vi "measure-tunnelling(SubVI).vi"(0 ".NET引用句柄输入":refnum<k24>, 1 "error":refnum<queue>, 5 "Timeout (20000 ms)":u32=20000, 7 "Resource In":refnum<visa-resource-name>, 9 "scan current":bool, 11 "error in (no error)":errorcluster, 12 "ch str":string) -> (4 "data":string[](array[string]), 8 "Numeric":sgl, 15 "error out":errorcluster)   [LabVIEW 2019]
uses:
  lib/QDInstrument.dll
  ppms-6621&2182-7001 tunnelling/Keithley 622x/Configure/Format/Typedefs/KE622x -- Optional Meas Elements.ctl
  ppms-6621&2182-7001 tunnelling/KE7001.LLB/Keith 7001 Open/Close Chan.vi
  ppms-6621&2182-7001 tunnelling/SubVI.lvlib
  ppms-6621&2182-7001 tunnelling/Keithley 622x/Keithley 622x.lvlib
panel:
  out "Timeout? 2":bool
  out "Execution Time 2":dbl
  out "array w/ subset deleted 2":sgl[](array[numeric])
  out "element 2":bool
  out "array w/ subset deleted":sgl[](array[numeric])
  out "element":bool
  out "Execution Time":dbl
  out "Timeout?":bool
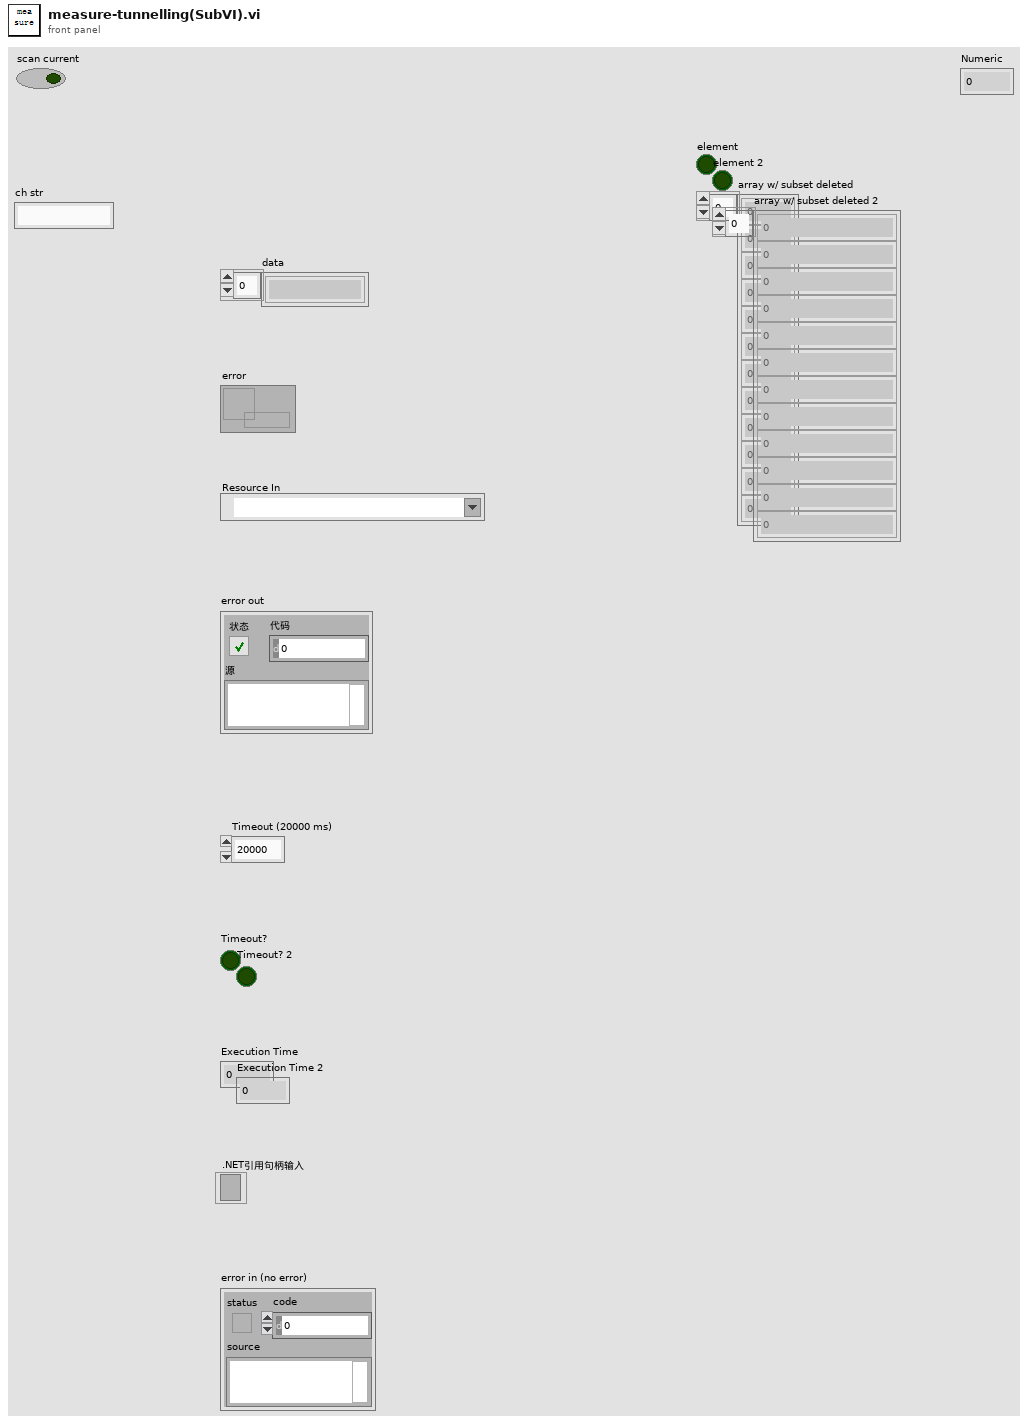
[diagram p1: front panel]
types:
  T1 = cluster{"slot/memory":i16, "channel/row":i16, "column":i16, bool, bool}[]
  T2 = typedef "Keithley 622x.lvlib/KE622x -- Optional Meas Elements.ctl" = cluster{"Timstamp?":bool, "Reading Num?":bool, "Source Value?":bool, "Compliance?":bool, "Average Voltage?":bool}
  T3 = cluster{"error":bool, "code":i32, "source":string}
  T4 = typedef "Keithley 622x.lvlib/KE622x -- Meas Event Reg State.ctl" = cluster{"B0, ROF:  KE2182A Delta Reading Overflow Event?":bool, "B1, Int:  Interlock OK Event?":bool, "B2, Temp:  Over Temperature Event?":bool, "B3, Comp:  Compliance Event?":bool, "B5, RAV:  Delta Reading Available Event?":bool, "B6, TN:  User Defined Reading Number Stored In Buffer Event?":bool, "B7, BAV:  At Least 2 Readings Stored In Buffer Event?":bool, "B12, BQF:  Buffer Quarter Full Event?":bool, "B8, BHF:  Buffer Half Full Event?":bool, "B13, B3QF:  Buffer 3/4 Full Event?":bool, "B9, BFL:  Buffer Full Event?":bool}
  T5 = typedef "Keithley 622x.lvlib/KE622x -- Trace Buf.ctl" = cluster{"Additional Valid Arrays":T2, "Reading Num":u32[], "Timestamp (secs)":sgl[], "Source Val (A)":sgl[], "Reading":sgl[], "Average Voltage (V)":sgl[], "Compliance?":bool[]}
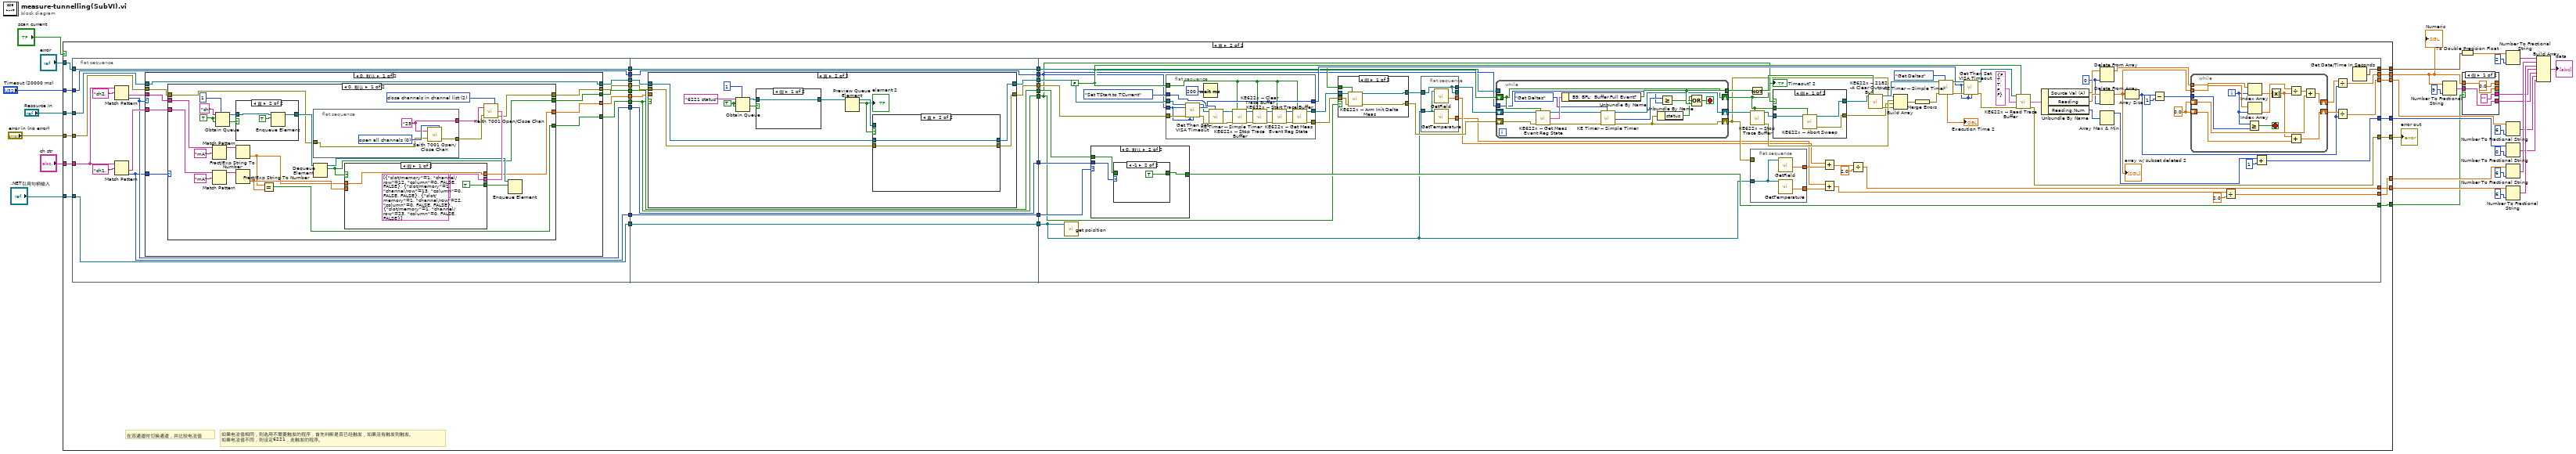
[diagram p0: block diagram]
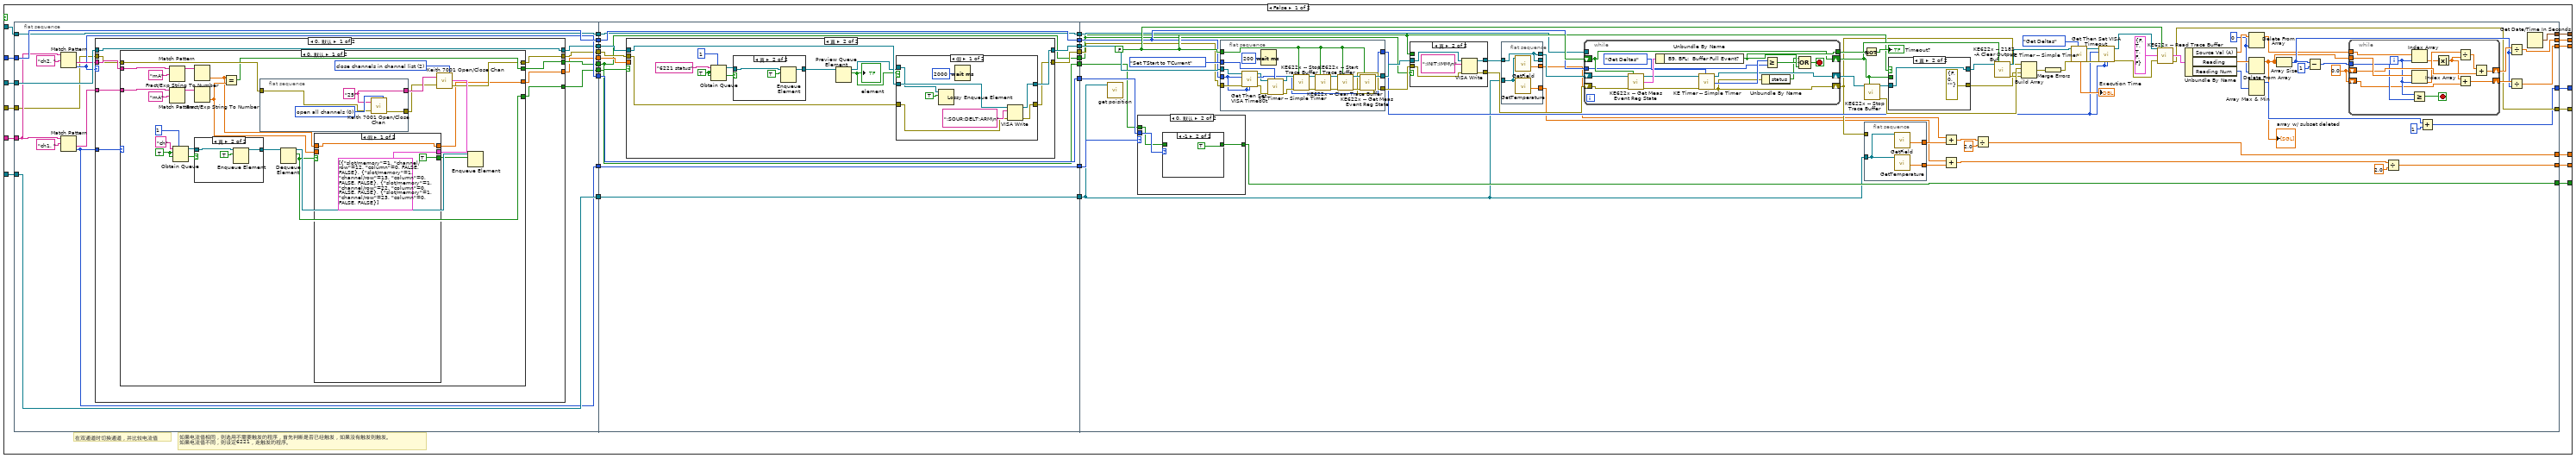
[diagram p2: hidden frame]
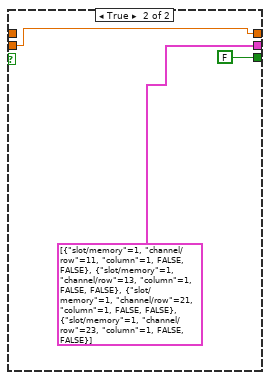
[diagram p4: hidden frame]
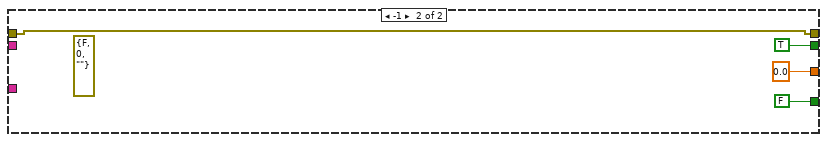
[diagram p5: hidden frame]
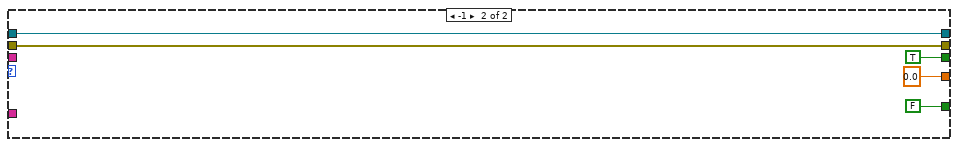
[diagram p6: hidden frame]
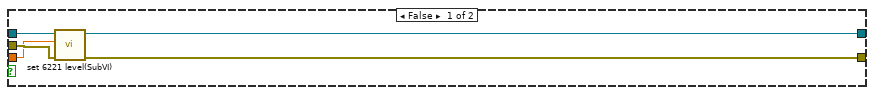
[diagram p7: hidden frame]
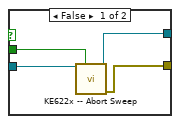
[diagram p10: hidden frame]
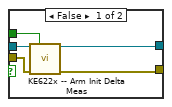
[diagram p11: hidden frame]
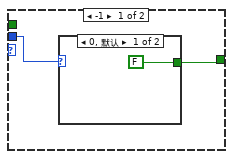
[diagram p12: hidden frame]
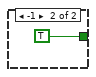
[diagram p13: hidden frame]
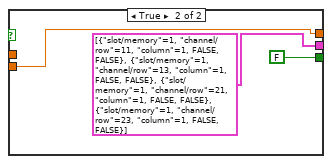
[diagram p16: hidden frame]
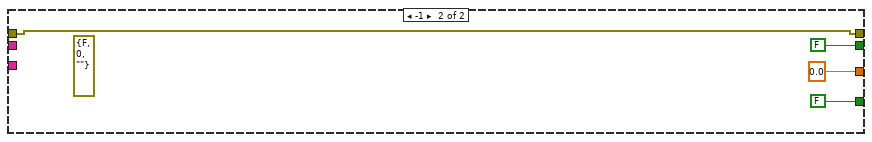
[diagram p17: hidden frame]
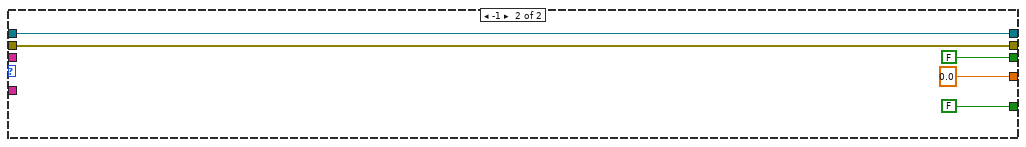
[diagram p18: hidden frame]
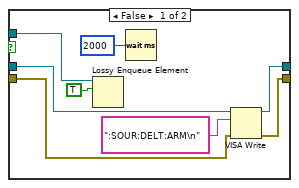
[diagram p20: hidden frame]
diagram:
  n1 = case shown="真" "scan current" {
    tunnel: [w45 w342] -> w31
    tunnel: ".NET引用句柄输入" -> [w44 w330]
    tunnel: "Resource In" -> [w43 w341]
    tunnel: "error in (no error)" -> [w42 w340]
    tunnel: "Timeout (20000 ms)" -> [w41 w339]
    tunnel: "error" -> [w40 w329]
    tunnel: [w39 w338] -> w25
    tunnel: [w38 w337] -> w22
    tunnel: [w37 w336] -> w19
    tunnel: [w36 w335] -> w9
    tunnel: "ch str" -> [w35 w334]
    tunnel: [w34 w333] -> w7
    tunnel: [w33 w332] -> w6
    tunnel: [w32 w331] -> w2
    frame False {
      # "如果电流值相同，则选用不需要触发的程序，首先判断是否已经触发，如果没有触发则触发。\n如果电流值不同，则设定6221，走触发的程序。"
      # "在双通道时切换通道，并比较电流值"
      n2 = flat-sequence {
        tunnel: w40 -> [w79]
        tunnel: w41 -> [w80]
        tunnel: w42 -> [w69]
        tunnel: w43 -> [w76]
        tunnel: w44 -> [w81]
        tunnel: [w81] -> w64
        tunnel: [w80] -> w63
        tunnel: [w79] -> w62
        tunnel: w35 -> [w75]
        tunnel: [w72] -> w61
        tunnel: [w71] -> w60
        tunnel: [w70] -> w59
        tunnel: [w68] -> w58
        tunnel: [w67] -> w57
        tunnel: [w66] -> w56
        tunnel: [w65] -> w55
        tunnel: w64 -> [w150]
        tunnel: [w150] -> w54
        tunnel: w63 -> [w149]
        tunnel: [w149] -> w53
        tunnel: w62 -> [w148]
        tunnel: [w148] -> w52
        tunnel: w61 -> [w147]
        tunnel: [w147] -> w51
        tunnel: w60 -> [w146]
        tunnel: [w146] -> w50
        tunnel: w59 -> [w145]
        tunnel: [w145] -> w49
        tunnel: w58 -> [w139]
        tunnel: w57 -> [w144]
        tunnel: w56 -> [w143]
        tunnel: w55 -> [w142]
        tunnel: [w141] -> w48
        tunnel: [w140] -> w47
        tunnel: [w139] -> w46
        tunnel: [w187] -> w38
        tunnel: [w188] -> w37
        tunnel: [w201] -> w45
        tunnel: [w224] -> w34
        tunnel: [w207] -> w36
        tunnel: [w219] -> w33
        tunnel: [w218] -> w39
        tunnel: w54 -> [w199]
        tunnel: w53 -> [w216]
        tunnel: w52 -> [w215]
        tunnel: [w206] -> w32
        tunnel: w51 -> [w205]
        tunnel: w50 -> [w204]
        tunnel: w49 -> [w203]
        tunnel: w48 -> [w217]
        tunnel: w47 -> [w228]
        tunnel: w46 -> [w202]
        frame #0 {
          n3 = Match Pattern(string=w75, regular expression="ch2, " ("正则表达式")) -> (after substring=w73:string, offset past match=w72:i32)  [unwired: 1 in, 2 out]
          n4 = Match Pattern(string=w75, regular expression="ch1, " ("正则表达式")) -> (after substring=w74:string, offset past match=w71:i32)  [unwired: 1 in, 2 out]
          n5 = case shown="0, 默认" w72 {
            tunnel: w76 -> [w82 w136]
            tunnel: w74 -> [w90 _]
            tunnel: w73 -> [w89 _]
            tunnel: w71 -> [w88 _]
            tunnel: [w87 FALSE ("create if not found? (T)")] -> w70
            tunnel: w69 -> [w86 w137]
            tunnel: [w85 TRUE] -> w68
            tunnel: [w84 w137] -> w67
            tunnel: [w83 0.0] -> w66
            tunnel: [w82 w136] -> w65
            frame 0, Default {
              n6 = case shown="0, 默认" w88 {
                tunnel: w90 -> [w101 _]
                tunnel: w89 -> [w111 _]
                tunnel: [w103 FALSE ("create if not found? (T)")] -> w87
                tunnel: w86 -> [w97 w131]
                tunnel: [w94 TRUE] -> w85
                tunnel: [w93 w131] -> w84
                tunnel: [w92 0.0] -> w83
                frame 0, Default {
                  w109 = TRUE ("create if not found? (T)")
                  w114 = u16 2 items=["open all channels", "open channels in channel list", "close channels in channel list"] ("open/close (open all:0)")
                  n7 = Match Pattern(string=w111, regular expression="mA" ("正则表达式")) -> (before substring=w98:string)  [unwired: 1 in, 3 out]
                  n8 = Match Pattern(string=w101, regular expression="mA" ("正则表达式")) -> (before substring=w99:string)  [unwired: 1 in, 3 out]
                  n9 = Obtain Queue(max queue size (-1, unlimited)=1, name (unnamed)="ch", element data type=w109, create if not found? (T)=w109) -> (queue out=w107:refnum<queue>, created new?=w108:bool)  [unwired: 1 in, 1 out]
                  n10 = Fract/Exp String To Number(string=w98) -> (number=w95:dbl)  [unwired: 3 in, 1 out]
                  n11 = Fract/Exp String To Number(string=w99) -> (number=w96:dbl)  [unwired: 3 in, 1 out]
                  n12 = case shown="真" w108 {
                    tunnel: w107 -> [w116 w119]
                    tunnel: [w116 w117] -> w106
                    frame False {
                    }
                    frame True {
                      n13 = Enqueue Element(queue=w119, element=TRUE) -> (queue out=w117:refnum<queue>)  [unwired: 2 in, 2 out]
                    }
                  }
                  n14 = Equal?(x=w95, y=w96) -> (x = y?=w94:bool)
                  n15 = flat-sequence {
                    tunnel: [w122] -> w115
                    tunnel: [w121] -> w112
                    tunnel: w97 -> [w120]
                    frame #0 {
                      w123 = u16 0 items=["open all channels", "open channels in channel list", "close channels in channel list"] ("open/close (open all:0)")
                      w122 = "25" ("GPIB address")
                      n16 = call "Keith 7001 Open/Close Chan.vi"("GPIB address"=w122, "error in"=w120, "open/close (open all:0)"=w123) -> ("error out"=w121:T3)  [unwired: 1 in]
                    }
                  }
                  n17 = Dequeue Element(queue=w106) -> (queue out=w105:refnum<queue>, element=w103:bool)  [unwired: 2 in, 2 out]
                  n18 = case shown="假" w103 {
                    tunnel: [T1 [{"slot/memory"=1, "channel/row"=12, "column"=0, FALSE, FALSE}, {"slot/memory"=1, "channel/row"=13, "column"=0, FALSE, FALSE}, {"slot/memory"=1, "channel/row"=22, "column"=0, FALSE, FALSE}, {"slot/memory"=1, "channel/row"=23, "column"=0, FALSE, FALSE}] ("channel list") T1 [{"slot/memory"=1, "channel/row"=11, "column"=1, FALSE, FALSE}, {"slot/memory"=1, "channel/row"=13, "column"=1, FALSE, FALSE}, {"slot/memory"=1, "channel/row"=21, "column"=1, FALSE, FALSE}, {"slot/memory"=1, "channel/row"=23, "column"=1, FALSE, FALSE}] ("channel list")] -> w113
                    tunnel: [TRUE FALSE] -> w104
                    tunnel: w96 -> [_ w128]
                    tunnel: w95 -> [w124 _]
                    tunnel: [w124 w128] -> w92
                    frame False {
                    }
                    frame True {
                    }
                  }
                  n19 = call "Keith 7001 Open/Close Chan.vi"("GPIB address"=w115, "error in"=w112, "open/close (open all:0)"=w114, "channel list"=w113) -> ("error out"=w93:T3)
                  n20 = Enqueue Element(queue=w105, element=w104) -> ()  [unwired: 2 in, 3 out]
                }
                frame -1 {
                  (unwired) errorcluster {"status"=FALSE, "code"=0, "source"=""} ("错误输出")
                }
              }
            }
            frame -1 {
            }
          }
        }
        frame #1 {
          n21 = case shown="真" w139 {
            tunnel: w144 -> [w155 w162]
            tunnel: w143 -> [w154 _]
            tunnel: w142 -> [w153 w163]
            tunnel: [w152 w161] -> w140
            tunnel: [w151 w160] -> w141
            frame False {
              n22 = call "set 6221 level(SubVI).vi"("错误输入（无错误）"=w155, "电流（mA）"=w154, "VISA引用句柄输入"=w153) -> ("错误输出"=w151:errorcluster, "VISA引用句柄输出"=w152:refnum<visa-resource-name>)  [unwired: 7 in]
            }
            frame True {
              w164 = TRUE ("create if not found? (T)")
              n23 = Obtain Queue(max queue size (-1, unlimited)=1, name (unnamed)="6221 status", element data type=w164, create if not found? (T)=w164) -> (queue out=w166:refnum<queue>, created new?=w167:bool)  [unwired: 1 in, 1 out]
              n24 = case shown="真" w167 {
                tunnel: w166 -> [w178 w181]
                tunnel: [w178 w179] -> w159
                frame False {
                }
                frame True {
                  n25 = Enqueue Element(queue=w181, element=TRUE) -> (queue out=w179:refnum<queue>)  [unwired: 2 in, 2 out]
                }
              }
              n26 = Preview Queue Element(queue=w159) -> (queue out=w158:refnum<queue>, element=w157:bool)  [unwired: 2 in, 2 out]
              "element" <- w157
              n27 = case shown="假" w157 {
                tunnel: w158 -> [w170 _]
                tunnel: w163 -> [w171 w176]
                tunnel: [w172 w176] -> w161
                tunnel: w162 -> [w174 w177]
                tunnel: [w173 w177] -> w160
                frame False {
                  n28 = Lossy Enqueue Element(queue=w170, element=TRUE) -> ()  [unwired: 1 in, 4 out]
                  n29 = Wait (ms)(milliseconds to wait=u32 2000) -> ()  [unwired: 1 out]
                  n30 = VISA Write(VISA resource name=w171, write buffer=":SOUR:DELT:ARM\n" ("format string"), error in (no error)=w174) -> (VISA resource name out=w172:refnum<visa-resource-name>, error out=w173:errorcluster)  [unwired: 1 out]
                }
                frame True {
                }
              }
            }
          }
        }
        frame #2 {
          w227 = FALSE ("Check For SCPI Errors? (T) 2")
          w184 = 0 ("index")
          w222 = sgl 0.0 ("Numeric")
          n31 = call "get poisition.vi"("Instrument Ref In"=w199) -> ()  [unwired: 4 in, 3 out]
          n32 = case shown="0, 默认" w204 {
            tunnel: [w293 w298] -> w206
            tunnel: w205 -> [w292 w297]
            tunnel: w203 -> [_ w296]
            frame -1 {
              n33 = case shown="0, 默认" w292 {
                tunnel: [FALSE TRUE] -> w293
                frame 0, Default {
                }
                frame -1 {
                }
              }
            }
            frame 0, Default {
              n34 = case shown="-1" w297 {
                tunnel: [w299 TRUE] -> w298
                tunnel: w296 -> [w299 _]
                frame 0, Default {
                }
                frame -1 {
                }
              }
            }
          }
          n35 = flat-sequence {
            tunnel: enum16{"Set TStart to TCurrent", "Get Deltas"}."Set TStart to TCurrent" ("Action") -> [w264]
            tunnel: [w261] -> w237
            tunnel: [w260] -> w236
            tunnel: [w257] -> w229
            tunnel: w228 -> [w254]
            tunnel: w227 -> [w253]
            tunnel: w217 -> [w252]
            tunnel: w216 -> [w251]
            frame #0 {
              n36 = call "Get Then Set VISA Timeout.vi"("VISA Resource Name In"=w254, "New Timeout (msecs)"=w251, "error in (no error)"=w252, "Max Timeout (300 secs)"=w251, "Min Timeout (3 secs)"=w251) -> ("VISA Resource Name Out (dupl)"=w256:refnum<visa-resource-name>, "Old Timeout (msecs)"=w257:u32, "error out"=w255:errorcluster)  [unwired: 7 in, 1 out]
              n37 = Wait (ms)(milliseconds to wait=u32 200) -> ()  [unwired: 1 out]
              n38 = call "KE Timer -- Simple Timer.vi"("Resource In"=w256, "error in (no error)"=w255, "Action"=w264) -> ("Resource Out (dupl)"=w263:refnum<visa-resource-name>, "error out (dupl)"=w262:errorcluster)  [unwired: 7 in, 8 out]
              n39 = call "KE622x -- Stop Trace Buffer.vi"("Resource In"=w263, "Check For SCPI Errors? (T)"=w253, "error in (no error)"=w262) -> ("Resource Out (dupl)"=w268:refnum<visa-resource-name>, "error out"=w267:errorcluster)  [unwired: 11 in]
              n40 = call "KE622x -- Clear Trace Buffer.vi"("Resource In"=w268, "Check For SCPI Errors? (T)"=w253, "error in (no error)"=w267) -> ("Resource Out (dupl)"=w259:refnum<visa-resource-name>, "error out"=w258:errorcluster)  [unwired: 11 in]
              n41 = call "KE622x -- Start Trace Buffer.vi"("Resource In"=w259, "Check For SCPI Errors? (T)"=w253, "error in (no error)"=w258) -> ("Resource Out (dupl)"=w265:refnum<visa-resource-name>, "error out"=w266:errorcluster)  [unwired: 11 in]
              n42 = call "KE622x -- Get Meas Event Reg State.vi"("VISA Resource In"=w265, "Error Query (T)?"=w253, "error in (no error)"=w266) -> ("VISA Resource Out (dupl)"=w261:refnum<visa-resource-name>, "error out"=w260:errorcluster)  [unwired: 10 in, 1 out]
            }
          }
          n43 = case shown="真" w202 {
            tunnel: [w286 w288] -> w244
            tunnel: [w285 w287] -> w198
            tunnel: w237 -> [w282 w290]
            tunnel: w236 -> [w284 w289]
            tunnel: w227 -> [w283 _]
            frame False {
              n44 = call "KE622x -- Arm Init Delta Meas.vi"("Resource In"=w282, "Check For SCPI Errors? (T)"=w283, "error in (no error)"=w284) -> ("Resource Out (dupl)"=w285:refnum<visa-resource-name>, "error out"=w286:errorcluster)  [unwired: 11 in]
            }
            frame True {
              n45 = VISA Write(VISA resource name=w290, write buffer=":INIT:IMM\n", error in (no error)=w289) -> (VISA resource name out=w287:refnum<visa-resource-name>, error out=w288:errorcluster)  [unwired: 1 out]
            }
          }
          n46 = flat-sequence {
            tunnel: w199 -> [w270]
            tunnel: [w272] -> w193
            tunnel: [w271] -> w196
            tunnel: w198 -> [w269]
            tunnel: [w269] -> _
            tunnel: [w269] -> w197
            frame #0 {
              n47 = call "GetField.vi"("Instrument Ref In"=w270) -> ("Field"=w271:dbl)  [unwired: 4 in, 4 out]
              n48 = call "GetTemperature.vi"("Instrument Ref In"=w270) -> ("Temperature"=w272:dbl)  [unwired: 4 in, 4 out]
            }
          }
          n49 = while {
            shift-right: [w303] -> w200
            shift-left: w244 -> [w315]
            shift-right: [w305] -> w241
            shift-left: w197 -> [w314]
            tunnel: [w307] -> w243
            shift-right: [w304] -> w213
            shift-left: w227 -> [w304]
            tunnel: w216 -> [w301]
            tunnel: w215 -> [_]
            stop <- w308 stop-if-true
            n50 = call "KE622x -- Get Meas Event Reg State.vi"("VISA Resource In"=w314, "Error Query (T)?"=w304, "error in (no error)"=w315) -> ("VISA Resource Out (dupl)"=w311:refnum<visa-resource-name>, "KE622x Meas Event Reg"=w313:T4, "error out"=w312:errorcluster)  [unwired: 10 in]
            n51 = Unbundle By Name(w313) -> ("B9, BFL:  Buffer Full Event?"=w307:bool)
            n52 = call "KE Timer -- Simple Timer.vi"("Resource In"=w311, "error in (no error)"=w312, "Action"=enum16{"Set TStart to TCurrent", "Get Deltas"}."Get Deltas") -> ("Resource Out (dupl)"=w305:refnum<visa-resource-name>, "TCurrent - TStart (ms)"=w309:u32, "error out (dupl)"=w303:errorcluster)  [unwired: 7 in, 7 out]
            n53 = Unbundle By Name(w303) -> ("status"=w302:bool)
            n54 = Greater Or Equal?(x=w309, y=w301) -> (x >= y?=w306:bool)
            n55 = Compound Arithmetic op=OR(w302, w306, w307) -> (w308:bool)
          }
          n56 = Not(x=w243) -> (.not. x?=→"Timeout?":bool)
          n57 = call "KE622x -- Stop Trace Buffer.vi"("Resource In"=w241, "Check For SCPI Errors? (T)"=w213) -> ("Resource Out (dupl)"=w214:refnum<visa-resource-name>, "error out"=w234:errorcluster)  [unwired: 12 in]
          n58 = flat-sequence {
            tunnel: w199 -> [w273]
            tunnel: [w275] -> w194
            tunnel: [w274] -> w195
            tunnel: w200 -> [_]
            frame #0 {
              n59 = call "GetField.vi"("Instrument Ref In"=w273) -> ("Field"=w274:dbl)  [unwired: 4 in, 4 out]
              n60 = call "GetTemperature.vi"("Instrument Ref In"=w273) -> ("Temperature"=w275:dbl)  [unwired: 4 in, 4 out]
            }
          }
          n61 = case shown="真" w202 {
            tunnel: w213 -> [w278 _]
            tunnel: [w277 w281] -> w212
            tunnel: [w276 errorcluster {"status"=FALSE, "code"=0, "source"=""} ("error out")] -> w211
            tunnel: w214 -> [w279 w281]
            frame False {
              n62 = call "KE622x -- Abort Sweep.vi"("Resource In"=w279, "Check For SCPI Errors? (T)"=w278) -> ("Resource Out (dupl)"=w277:refnum<visa-resource-name>, "error out"=w276:errorcluster)  [unwired: 12 in]
            }
            frame True {
            }
          }
          n63 = Add(x=w196, y=w195) -> (x+y=w191:dbl)
          n64 = Add(x=w193, y=w194) -> (x+y=w192:dbl)
          n65 = Divide(x=w191, y=2.0) -> (x/y=w188:dbl)
          n66 = call "KE622x -- 2182 -A Clear Output Buf.vi"("622x Resource In"=w212, "Check For SCPI Errors? (T)"=w213) -> ("622x Resource Out (dupl)"=w240:refnum<visa-resource-name>, "error out"=w233:errorcluster)  [unwired: 11 in, 1 out]
          n67 = Build Array(w200, w234, w211, w233) -> (w235:errorcluster[])
          n68 = Merge Errors(w235) -> (w232:errorcluster)
          n69 = call "KE Timer -- Simple Timer.vi"("Resource In"=w240, "error in (no error)"=w232, "Action"=enum16{"Set TStart to TCurrent", "Get Deltas"}."Get Deltas") -> ("TCurrent - TStart (s)"=→"Execution Time":dbl, "Resource Out (dupl)"=w230:refnum<visa-resource-name>, "error out (dupl)"=w231:errorcluster)  [unwired: 7 in, 7 out]
          n70 = call "Get Then Set VISA Timeout.vi"("VISA Resource Name In"=w230, "New Timeout (msecs)"=w229, "error in (no error)"=w231, "Max Timeout (300 secs)"=w229, "Min Timeout (3 secs)"=w229) -> ("VISA Resource Name Out (dupl)"=w226:refnum<visa-resource-name>, "error out"=w225:errorcluster)  [unwired: 7 in, 2 out]
          n71 = call "KE622x -- Read Trace Buffer.vi"("Resource In"=w226, "Check For SCPI Errors? (T)"=w227, "Meas Elements To Return"=T2 {"Timstamp?"=FALSE, "Reading Num?"=TRUE, "Source Value?"=TRUE, "Compliance?"=FALSE, "Average Voltage?"=FALSE}, "error in (no error)"=w225) -> ("Trace Buf"=w249:T5, "error out"=w218:errorcluster)  [unwired: 9 in, 1 out]
          n72 = Unbundle By Name(w249) -> ("Source Val (A)"=w185:sgl[], "Reading"=w186:sgl[], "Reading Num"=w223:u32[])
          n73 = Delete From Array(array=w185, index=w184) -> (array with subset deleted=w183:sgl[])  [unwired: 1 in, 1 out]
          n74 = Delete From Array(array=w186, index=w184) -> (array with subset deleted=w182:sgl[])  [unwired: 1 in, 1 out]
          "array w/ subset deleted" <- w182
          n75 = Array Max & Min(array=w223) -> (max value=w209:u32)  [unwired: 3 out]
          n76 = Array Size(array=w182) -> (size(s)=w220:i32)
          n77 = Subtract(x=w220, y=1) -> (x-y=w246:i32)
          n78 = while {
            tunnel: w182 -> [w328]
            shift-right: [w326] -> w248
            shift-left: w222 -> [w327]
            tunnel: w246 -> [w325]
            tunnel: w183 -> [w323]
            shift-right: [w320] -> w221
            shift-left: w222 -> [w321]
            i -> [w322]
            stop <- w324 stop-if-true
            n79 = Greater Or Equal?(x=w322, y=w325) -> (x >= y?=w324:bool)
            n80 = Index Array(array=w323, index=w322) -> (element=w318:sgl)
            n81 = Index Array(array=w328, index=w322) -> (element=w319:sgl)
            n82 = Absolute Value(x=w318) -> (abs(x)=w316:sgl)
            n83 = Divide(x=w319, y=w316) -> (x/y=w317:sgl)
            n84 = Add(x=w316, y=w321) -> (x+y=w320:sgl)
            n85 = Add(x=w317, y=w327) -> (x+y=w326:sgl)
          }
          n86 = Divide(x=w192, y=2.0) -> (x/y=w187:dbl)
          n87 = Add(x=w209, y=u32 1) -> (x+y=w207:u32)
          n88 = Divide(x=w248, y=w220) -> (x/y=w224:sgl)
          n89 = Divide(x=w221, y=w220) -> (x/y=w219:sgl)
          n90 = Get Date/Time In Seconds() -> (seconds since 1Jan1904=w201:timestamp)
        }
      }
    }
    frame True {
      # "如果电流值相同，则选用不需要触发的程序，首先判断是否已经触发，如果没有触发则触发。\n如果电流值不同，则设定6221，走触发的程序。"
      # "在双通道时切换通道，并比较电流值"
      n91 = flat-sequence {
        tunnel: w329 -> [w376]
        tunnel: w339 -> [w377]
        tunnel: w340 -> [w366]
        tunnel: w341 -> [w373]
        tunnel: w330 -> [w378]
        tunnel: [w378] -> w361
        tunnel: [w377] -> w360
        tunnel: [w376] -> w359
        tunnel: w334 -> [w372]
        tunnel: [w369] -> w358
        tunnel: [w368] -> w357
        tunnel: [w367] -> w356
        tunnel: [w365] -> w355
        tunnel: [w364] -> w354
        tunnel: [w363] -> w353
        tunnel: [w362] -> w352
        tunnel: w361 -> [w447]
        tunnel: [w447] -> w351
        tunnel: w360 -> [w446]
        tunnel: [w446] -> w350
        tunnel: w359 -> [w445]
        tunnel: [w445] -> w349
        tunnel: w358 -> [w444]
        tunnel: [w444] -> w348
        tunnel: w357 -> [w443]
        tunnel: [w443] -> w347
        tunnel: w356 -> [w442]
        tunnel: [w442] -> w346
        tunnel: w355 -> [w436]
        tunnel: w354 -> [w441]
        tunnel: w353 -> [w440]
        tunnel: w352 -> [w439]
        tunnel: [w438] -> w345
        tunnel: [w437] -> w344
        tunnel: [w436] -> w343
        tunnel: [w481] -> w337
        tunnel: [w482] -> w336
        tunnel: [w495] -> w342
        tunnel: [w518] -> w333
        tunnel: [w501] -> w335
        tunnel: [w513] -> w332
        tunnel: [w512] -> w338
        tunnel: w351 -> [w493]
        tunnel: w350 -> [w510]
        tunnel: w349 -> [w509]
        tunnel: [w500] -> w331
        tunnel: w348 -> [w499]
        tunnel: w347 -> [w498]
        tunnel: w346 -> [w497]
        tunnel: w345 -> [w511]
        tunnel: w344 -> [w522]
        tunnel: w343 -> [w496]
        frame #0 {
          n92 = Match Pattern(string=w372, regular expression="ch2, " ("正则表达式")) -> (after substring=w370:string, offset past match=w369:i32)  [unwired: 1 in, 2 out]
          n93 = Match Pattern(string=w372, regular expression="ch1, " ("正则表达式")) -> (after substring=w371:string, offset past match=w368:i32)  [unwired: 1 in, 2 out]
          n94 = case shown="0, 默认" w369 {
            tunnel: w373 -> [w379 w433]
            tunnel: w371 -> [w387 _]
            tunnel: w370 -> [w386 _]
            tunnel: w368 -> [w385 _]
            tunnel: [w384 FALSE ("create if not found? (T)")] -> w367
            tunnel: w366 -> [w383 w434]
            tunnel: [w382 FALSE] -> w365
            tunnel: [w381 w434] -> w364
            tunnel: [w380 0.0] -> w363
            tunnel: [w379 w433] -> w362
            frame 0, Default {
              n95 = case shown="0, 默认" w385 {
                tunnel: w387 -> [w398 _]
                tunnel: w386 -> [w408 _]
                tunnel: [w400 FALSE ("create if not found? (T)")] -> w384
                tunnel: w383 -> [w394 w428]
                tunnel: [w391 FALSE] -> w382
                tunnel: [w390 w428] -> w381
                tunnel: [w389 0.0] -> w380
                frame 0, Default {
                  w406 = TRUE ("create if not found? (T)")
                  w411 = u16 2 items=["open all channels", "open channels in channel list", "close channels in channel list"] ("open/close (open all:0)")
                  n96 = Match Pattern(string=w408, regular expression="mA" ("正则表达式")) -> (before substring=w395:string)  [unwired: 1 in, 3 out]
                  n97 = Match Pattern(string=w398, regular expression="mA" ("正则表达式")) -> (before substring=w396:string)  [unwired: 1 in, 3 out]
                  n98 = Obtain Queue(max queue size (-1, unlimited)=1, name (unnamed)="ch", element data type=w406, create if not found? (T)=w406) -> (queue out=w404:refnum<queue>, created new?=w405:bool)  [unwired: 1 in, 1 out]
                  n99 = case shown="真" w405 {
                    tunnel: w404 -> [w413 w416]
                    tunnel: [w413 w414] -> w403
                    frame False {
                    }
                    frame True {
                      n100 = Enqueue Element(queue=w416, element=TRUE) -> (queue out=w414:refnum<queue>)  [unwired: 2 in, 2 out]
                    }
                  }
                  n101 = Fract/Exp String To Number(string=w395) -> (number=w392:dbl)  [unwired: 3 in, 1 out]
                  n102 = Fract/Exp String To Number(string=w396) -> (number=w393:dbl)  [unwired: 3 in, 1 out]
                  n103 = Equal?(x=w392, y=w393) -> (x = y?=w391:bool)
                  n104 = flat-sequence {
                    tunnel: [w419] -> w412
                    tunnel: [w418] -> w409
                    tunnel: w394 -> [w417]
                    frame #0 {
                      w420 = u16 0 items=["open all channels", "open channels in channel list", "close channels in channel list"] ("open/close (open all:0)")
                      w419 = "25" ("GPIB address")
                      n105 = call "Keith 7001 Open/Close Chan.vi"("GPIB address"=w419, "error in"=w417, "open/close (open all:0)"=w420) -> ("error out"=w418:T3)  [unwired: 1 in]
                    }
                  }
                  n106 = Dequeue Element(queue=w403) -> (queue out=w402:refnum<queue>, element=w400:bool)  [unwired: 2 in, 2 out]
                  n107 = case shown="假" w400 {
                    tunnel: [T1 [{"slot/memory"=1, "channel/row"=12, "column"=0, FALSE, FALSE}, {"slot/memory"=1, "channel/row"=13, "column"=0, FALSE, FALSE}, {"slot/memory"=1, "channel/row"=22, "column"=0, FALSE, FALSE}, {"slot/memory"=1, "channel/row"=23, "column"=0, FALSE, FALSE}] ("channel list") T1 [{"slot/memory"=1, "channel/row"=11, "column"=1, FALSE, FALSE}, {"slot/memory"=1, "channel/row"=13, "column"=1, FALSE, FALSE}, {"slot/memory"=1, "channel/row"=21, "column"=1, FALSE, FALSE}, {"slot/memory"=1, "channel/row"=23, "column"=1, FALSE, FALSE}] ("channel list")] -> w410
                    tunnel: [TRUE FALSE] -> w401
                    tunnel: w393 -> [_ w424]
                    tunnel: w392 -> [w421 _]
                    tunnel: [w421 w424] -> w389
                    frame False {
                    }
                    frame True {
                    }
                  }
                  n108 = call "Keith 7001 Open/Close Chan.vi"("GPIB address"=w412, "error in"=w409, "open/close (open all:0)"=w411, "channel list"=w410) -> ("error out"=w390:T3)
                  n109 = Enqueue Element(queue=w402, element=w401) -> ()  [unwired: 2 in, 3 out]
                }
                frame -1 {
                  (unwired) errorcluster {"status"=FALSE, "code"=0, "source"=""} ("错误输出")
                }
              }
            }
            frame -1 {
            }
          }
        }
        frame #1 {
          n110 = case shown="真" w436 {
            tunnel: w441 -> [w448 w456]
            tunnel: w440 -> [_ _]
            tunnel: w439 -> [w449 w457]
            tunnel: [w449 w455] -> w437
            tunnel: [w448 w454] -> w438
            frame False {
            }
            frame True {
              w458 = TRUE ("create if not found? (T)")
              n111 = Obtain Queue(max queue size (-1, unlimited)=1, name (unnamed)="6221 status", element data type=w458, create if not found? (T)=w458) -> (queue out=w460:refnum<queue>, created new?=w461:bool)  [unwired: 1 in, 1 out]
              n112 = case shown="假" w461 {
                tunnel: w460 -> [w472 w475]
                tunnel: [w472 w473] -> w453
                frame False {
                }
                frame True {
                  n113 = Enqueue Element(queue=w475, element=TRUE) -> (queue out=w473:refnum<queue>)  [unwired: 2 in, 2 out]
                }
              }
              n114 = Preview Queue Element(queue=w453) -> (queue out=w452:refnum<queue>, element=w451:bool)  [unwired: 2 in, 2 out]
              "element 2" <- w451
              n115 = case shown="真" w451 {
                tunnel: w452 -> [w464 _]
                tunnel: w457 -> [w465 w470]
                tunnel: [w466 w470] -> w455
                tunnel: w456 -> [w468 w471]
                tunnel: [w467 w471] -> w454
                frame False {
                  n116 = Lossy Enqueue Element(queue=w464, element=TRUE) -> ()  [unwired: 1 in, 4 out]
                  n117 = Wait (ms)(milliseconds to wait=u32 2000) -> ()  [unwired: 1 out]
                  n118 = VISA Write(VISA resource name=w465, write buffer=":SOUR:DELT:ARM\n" ("format string"), error in (no error)=w468) -> (VISA resource name out=w466:refnum<visa-resource-name>, error out=w467:errorcluster)  [unwired: 1 out]
                }
                frame True {
                }
              }
            }
          }
        }
        frame #2 {
          w521 = FALSE ("Check For SCPI Errors? (T) 3")
          w478 = 0 ("index")
          w516 = sgl 0.0 ("Numeric")
          n119 = call "get poisition.vi"("Instrument Ref In"=w493) -> ()  [unwired: 4 in, 3 out]
          n120 = case shown="0, 默认" w498 {
            tunnel: [w587 w592] -> w500
            tunnel: w499 -> [w586 w591]
            tunnel: w497 -> [_ w590]
            frame -1 {
              n121 = case shown="0, 默认" w586 {
                tunnel: [FALSE TRUE] -> w587
                frame 0, Default {
                }
                frame -1 {
                }
              }
            }
            frame 0, Default {
              n122 = case shown="-1" w591 {
                tunnel: [w593 TRUE] -> w592
                tunnel: w590 -> [w593 _]
                frame 0, Default {
                }
                frame -1 {
                }
              }
            }
          }
          n123 = flat-sequence {
            tunnel: enum16{"Set TStart to TCurrent", "Get Deltas"}."Set TStart to TCurrent" ("Action") -> [w558]
            tunnel: [w555] -> w531
            tunnel: [w554] -> w530
            tunnel: [w551] -> w523
            tunnel: w522 -> [w548]
            tunnel: w521 -> [w547]
            tunnel: w511 -> [w546]
            tunnel: w510 -> [w545]
            frame #0 {
              n124 = call "Get Then Set VISA Timeout.vi"("VISA Resource Name In"=w548, "New Timeout (msecs)"=w545, "error in (no error)"=w546, "Max Timeout (300 secs)"=w545, "Min Timeout (3 secs)"=w545) -> ("VISA Resource Name Out (dupl)"=w550:refnum<visa-resource-name>, "Old Timeout (msecs)"=w551:u32, "error out"=w549:errorcluster)  [unwired: 7 in, 1 out]
              n125 = Wait (ms)(milliseconds to wait=u32 200) -> ()  [unwired: 1 out]
              n126 = call "KE Timer -- Simple Timer.vi"("Resource In"=w550, "error in (no error)"=w549, "Action"=w558) -> ("Resource Out (dupl)"=w557:refnum<visa-resource-name>, "error out (dupl)"=w556:errorcluster)  [unwired: 7 in, 8 out]
              n127 = call "KE622x -- Stop Trace Buffer.vi"("Resource In"=w557, "Check For SCPI Errors? (T)"=w547, "error in (no error)"=w556) -> ("Resource Out (dupl)"=w562:refnum<visa-resource-name>, "error out"=w561:errorcluster)  [unwired: 11 in]
              n128 = call "KE622x -- Clear Trace Buffer.vi"("Resource In"=w562, "Check For SCPI Errors? (T)"=w547, "error in (no error)"=w561) -> ("Resource Out (dupl)"=w553:refnum<visa-resource-name>, "error out"=w552:errorcluster)  [unwired: 11 in]
              n129 = call "KE622x -- Start Trace Buffer.vi"("Resource In"=w553, "Check For SCPI Errors? (T)"=w547, "error in (no error)"=w552) -> ("Resource Out (dupl)"=w559:refnum<visa-resource-name>, "error out"=w560:errorcluster)  [unwired: 11 in]
              n130 = call "KE622x -- Get Meas Event Reg State.vi"("VISA Resource In"=w559, "Error Query (T)?"=w547, "error in (no error)"=w560) -> ("VISA Resource Out (dupl)"=w555:refnum<visa-resource-name>, "error out"=w554:errorcluster)  [unwired: 10 in, 1 out]
            }
          }
          n131 = case shown="假" w496 {
            tunnel: [w580 w582] -> w538
            tunnel: [w579 w581] -> w492
            tunnel: w531 -> [w576 w584]
            tunnel: w530 -> [w578 w583]
            tunnel: w521 -> [w577 _]
            frame False {
              n132 = call "KE622x -- Arm Init Delta Meas.vi"("Resource In"=w576, "Check For SCPI Errors? (T)"=w577, "error in (no error)"=w578) -> ("Resource Out (dupl)"=w579:refnum<visa-resource-name>, "error out"=w580:errorcluster)  [unwired: 11 in]
            }
            frame True {
              n133 = VISA Write(VISA resource name=w584, write buffer=":INIT:IMM\n", error in (no error)=w583) -> (VISA resource name out=w581:refnum<visa-resource-name>, error out=w582:errorcluster)  [unwired: 1 out]
            }
          }
          n134 = flat-sequence {
            tunnel: w493 -> [w564]
            tunnel: [w566] -> w487
            tunnel: [w565] -> w490
            tunnel: w492 -> [w563]
            tunnel: [w563] -> _
            tunnel: [w563] -> w491
            frame #0 {
              n135 = call "GetField.vi"("Instrument Ref In"=w564) -> ("Field"=w565:dbl)  [unwired: 4 in, 4 out]
              n136 = call "GetTemperature.vi"("Instrument Ref In"=w564) -> ("Temperature"=w566:dbl)  [unwired: 4 in, 4 out]
            }
          }
          n137 = while {
            shift-right: [w597] -> w494
            shift-left: w538 -> [w609]
            shift-right: [w599] -> w535
            shift-left: w491 -> [w608]
            tunnel: [w601] -> w537
            shift-right: [w598] -> w507
            shift-left: w521 -> [w598]
            tunnel: w510 -> [w595]
            tunnel: w509 -> [_]
            stop <- w602 stop-if-true
            n138 = call "KE622x -- Get Meas Event Reg State.vi"("VISA Resource In"=w608, "Error Query (T)?"=w598, "error in (no error)"=w609) -> ("VISA Resource Out (dupl)"=w605:refnum<visa-resource-name>, "KE622x Meas Event Reg"=w607:T4, "error out"=w606:errorcluster)  [unwired: 10 in]
            n139 = Unbundle By Name(w607) -> ("B9, BFL:  Buffer Full Event?"=w601:bool)
            n140 = call "KE Timer -- Simple Timer.vi"("Resource In"=w605, "error in (no error)"=w606, "Action"=enum16{"Set TStart to TCurrent", "Get Deltas"}."Get Deltas") -> ("Resource Out (dupl)"=w599:refnum<visa-resource-name>, "TCurrent - TStart (ms)"=w603:u32, "error out (dupl)"=w597:errorcluster)  [unwired: 7 in, 7 out]
            n141 = Unbundle By Name(w597) -> ("status"=w596:bool)
            n142 = Greater Or Equal?(x=w603, y=w595) -> (x >= y?=w600:bool)
            n143 = Compound Arithmetic op=OR(w596, w600, w601) -> (w602:bool)
          }
          n144 = Not(x=w537) -> (.not. x?=→"Timeout? 2":bool)
          n145 = call "KE622x -- Stop Trace Buffer.vi"("Resource In"=w535, "Check For SCPI Errors? (T)"=w507) -> ("Resource Out (dupl)"=w508:refnum<visa-resource-name>, "error out"=w528:errorcluster)  [unwired: 12 in]
          n146 = flat-sequence {
            tunnel: w493 -> [w567]
            tunnel: [w569] -> w488
            tunnel: [w568] -> w489
            tunnel: w494 -> [_]
            frame #0 {
              n147 = call "GetField.vi"("Instrument Ref In"=w567) -> ("Field"=w568:dbl)  [unwired: 4 in, 4 out]
              n148 = call "GetTemperature.vi"("Instrument Ref In"=w567) -> ("Temperature"=w569:dbl)  [unwired: 4 in, 4 out]
            }
          }
          n149 = case shown="假" w496 {
            tunnel: w507 -> [w572 _]
            tunnel: [w571 w575] -> w506
            tunnel: [w570 errorcluster {"status"=FALSE, "code"=0, "source"=""} ("error out")] -> w505
            tunnel: w508 -> [w573 w575]
            frame False {
              n150 = call "KE622x -- Abort Sweep.vi"("Resource In"=w573, "Check For SCPI Errors? (T)"=w572) -> ("Resource Out (dupl)"=w571:refnum<visa-resource-name>, "error out"=w570:errorcluster)  [unwired: 12 in]
            }
            frame True {
            }
          }
          n151 = Add(x=w490, y=w489) -> (x+y=w485:dbl)
          n152 = Add(x=w487, y=w488) -> (x+y=w486:dbl)
          n153 = Divide(x=w485, y=2.0) -> (x/y=w482:dbl)
          n154 = call "KE622x -- 2182 -A Clear Output Buf.vi"("622x Resource In"=w506, "Check For SCPI Errors? (T)"=w507) -> ("622x Resource Out (dupl)"=w534:refnum<visa-resource-name>, "error out"=w527:errorcluster)  [unwired: 11 in, 1 out]
          n155 = Build Array(w494, w528, w505, w527) -> (w529:errorcluster[])
          n156 = Merge Errors(w529) -> (w526:errorcluster)
          n157 = call "KE Timer -- Simple Timer.vi"("Resource In"=w534, "error in (no error)"=w526, "Action"=enum16{"Set TStart to TCurrent", "Get Deltas"}."Get Deltas") -> ("TCurrent - TStart (s)"=→"Execution Time 2":dbl, "Resource Out (dupl)"=w524:refnum<visa-resource-name>, "error out (dupl)"=w525:errorcluster)  [unwired: 7 in, 7 out]
          n158 = call "Get Then Set VISA Timeout.vi"("VISA Resource Name In"=w524, "New Timeout (msecs)"=w523, "error in (no error)"=w525, "Max Timeout (300 secs)"=w523, "Min Timeout (3 secs)"=w523) -> ("VISA Resource Name Out (dupl)"=w520:refnum<visa-resource-name>, "error out"=w519:errorcluster)  [unwired: 7 in, 2 out]
          n159 = call "KE622x -- Read Trace Buffer.vi"("Resource In"=w520, "Check For SCPI Errors? (T)"=w521, "Meas Elements To Return"=T2 {"Timstamp?"=FALSE, "Reading Num?"=TRUE, "Source Value?"=TRUE, "Compliance?"=FALSE, "Average Voltage?"=FALSE}, "error in (no error)"=w519) -> ("Trace Buf"=w543:T5, "error out"=w512:errorcluster)  [unwired: 9 in, 1 out]
          n160 = Unbundle By Name(w543) -> ("Source Val (A)"=w479:sgl[], "Reading"=w480:sgl[], "Reading Num"=w517:u32[])
          n161 = Delete From Array(array=w479, index=w478) -> (array with subset deleted=w477:sgl[])  [unwired: 1 in, 1 out]
          n162 = Delete From Array(array=w480, index=w478) -> (array with subset deleted=w476:sgl[])  [unwired: 1 in, 1 out]
          "array w/ subset deleted 2" <- w476
          n163 = Array Max & Min(array=w517) -> (max value=w503:u32)  [unwired: 3 out]
          n164 = Array Size(array=w476) -> (size(s)=w514:i32)
          n165 = Subtract(x=w514, y=1) -> (x-y=w540:i32)
          n166 = while {
            tunnel: w476 -> [w622]
            shift-right: [w620] -> w542
            shift-left: w516 -> [w621]
            tunnel: w540 -> [w619]
            tunnel: w477 -> [w617]
            shift-right: [w614] -> w515
            shift-left: w516 -> [w615]
            i -> [w616]
            stop <- w618 stop-if-true
            n167 = Greater Or Equal?(x=w616, y=w619) -> (x >= y?=w618:bool)
            n168 = Index Array(array=w617, index=w616) -> (element=w612:sgl)
            n169 = Index Array(array=w622, index=w616) -> (element=w613:sgl)
            n170 = Absolute Value(x=w612) -> (abs(x)=w610:sgl)
            n171 = Divide(x=w613, y=w610) -> (x/y=w611:sgl)
            n172 = Add(x=w610, y=w615) -> (x+y=w614:sgl)
            n173 = Add(x=w611, y=w621) -> (x+y=w620:sgl)
          }
          n174 = Divide(x=w486, y=2.0) -> (x/y=w481:dbl)
          n175 = Add(x=w503, y=u32 1) -> (x+y=w501:u32)
          n176 = Divide(x=w542, y=w514) -> (x/y=w518:sgl)
          n177 = Divide(x=w515, y=w514) -> (x/y=w513:sgl)
          n178 = Get Date/Time In Seconds() -> (seconds since 1Jan1904=w495:timestamp)
        }
      }
    }
  }
  "error out" <- w25
  "Numeric" <- w7
  n179 = Number To Fractional String(number=w7, precision (6)=i16 9 ("精度(6)")) -> (F-format string=w14:string)  [unwired: 2 in]
  n180 = To Double Precision Float(number=w31) -> (double precision float=w24:dbl)
  n181 = case shown="假" w2 {
    tunnel: [sgl 0.0 w630] -> _
    tunnel: w7 -> [w626 w630]
    tunnel: [w626 0.0 ("元素")] -> _
    tunnel: w14 -> [w623 w628]
    tunnel: ["" w628] -> w13
    tunnel: [w623 ""] -> w12
    frame False {
    }
    frame True {
    }
  }
  n182 = Number To Fractional String(number=w24, precision (6)=i16 2 ("精度(6)")) -> (F-format string=w17:string)  [unwired: 2 in]
  n183 = Number To Fractional String(number=w6, precision (6)=i16 6) -> (F-format string=w3:string)  [unwired: 2 in]
  n184 = Number To Fractional String(number=w9, precision (6)=i16 0 ("精度(6)")) -> (F-format string=w4:string)  [unwired: 2 in]
  n185 = Number To Fractional String(number=w19, precision (6)=i16 6 ("精度(6)")) -> (F-format string=w18:string)  [unwired: 2 in]
  n186 = Number To Fractional String(number=w22, precision (6)=i16 6 ("精度(6)")) -> (F-format string=w16:string)  [unwired: 2 in]
  n187 = Build Array(w17, w18, w16, w13, w12, w3, w4) -> (→"data":string[])
